vi "Pose2D_publisher.vi"() -> ()   [LabVIEW 2014]
panel:
  in  "cmdvel":T1={"msg.x"=1.01, "msg.y"=0.0, "msg.theta"=0.0}
  in  "停止":bool
  in  "发送":bool
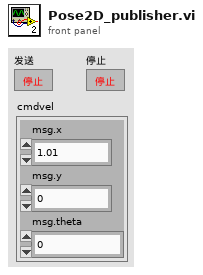
[diagram p1: front panel]
types:
  T1 = cluster{"msg.x":dbl, "msg.y":dbl, "msg.theta":dbl}
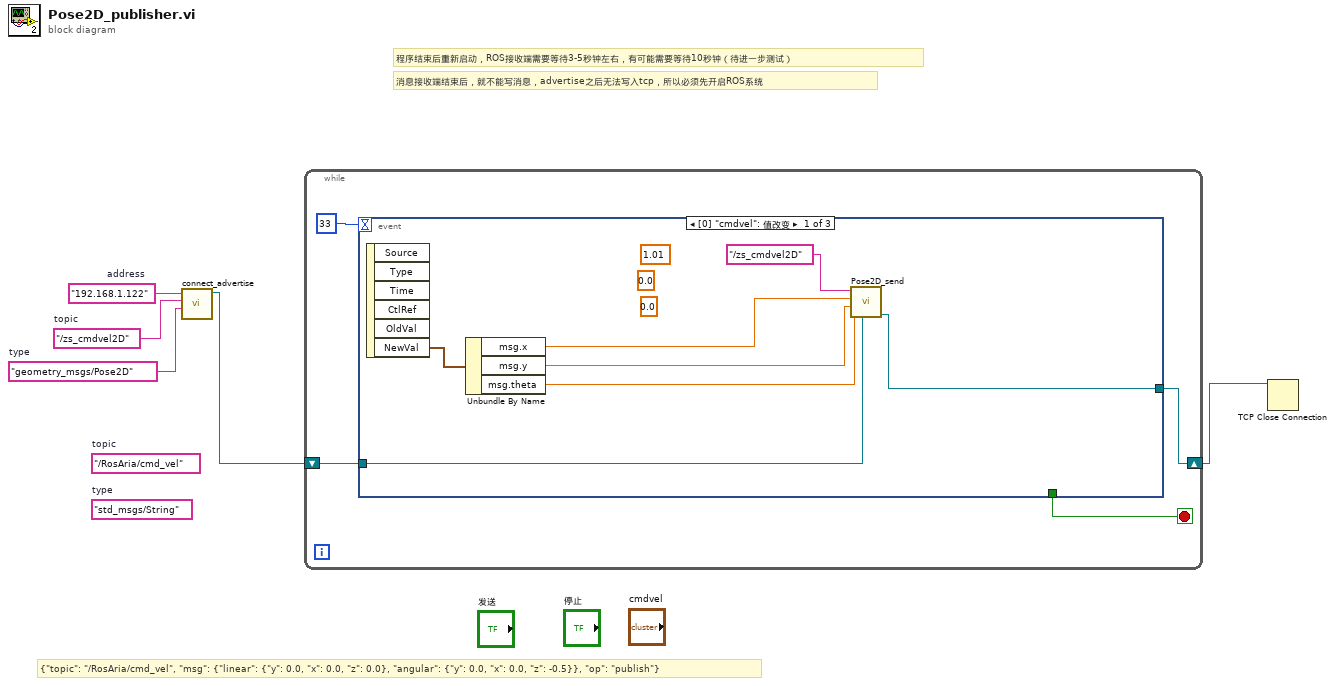
[diagram p0: block diagram]
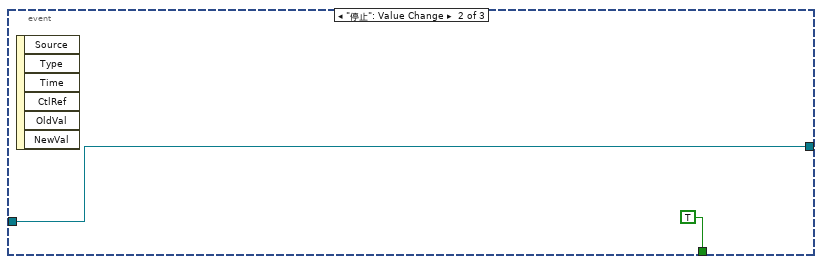
[diagram p2: hidden frame]
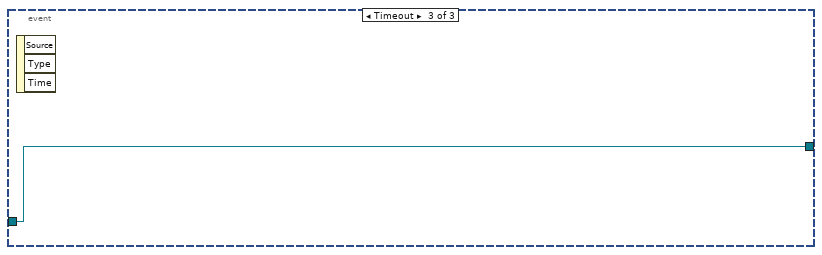
[diagram p3: hidden frame]
diagram:
  w4 = "192.168.1.122"  # address
  (unwired) "std_msgs/String"  # type
  w3 = "/zs_cmdvel2D"  # topic
  w1 = "geometry_msgs/Pose2D"  # type
  (unwired) "/RosAria/cmd_vel"  # topic
  # "消息接收端结束后，就不能写消息，advertise之后无法写入tcp，所以必须先开启ROS系统"
  # "{\"topic\": \"/RosAria/cmd_vel\", \"msg\": {\"linear\": {\"y\": 0.0, \"x\": 0.0, \"z\": 0.0}, \"angular\": {\"y\": 0.0, \"x\": 0.0, \"z\": -0.5}}, \"op\": \"publish\"}"
  # "程序结束后重新启动，ROS接收端需要等待3-5秒钟左右，有可能需要等待10秒钟（待进一步测试）"
  n1 = call "connect_advertise.vi"("type"=w1, "topic"=w3, "address"=w4) -> ("连接ID输出"=w2:refnum<k5>)  [unwired: 7 in, 1 out]
  n2 = while {
    shift-right: [w7] -> w5
    shift-left: w2 -> [w6]
    stop <- w8 stop-if-true
    n3 = event shown="[0] \"cmdvel\": 值改变" {
      selector: _ -> [_ _ _]
      dyn-events: _ -> [_ _ _]
      timeout: 33 -> [_ _ _]
      tunnel: [_ TRUE _] -> w8
      tunnel: [w10 w17 w19] -> w7
      tunnel: w6 -> [w16 w17 w19]
      event "cmdvel": Value Change {
        (unwired) 0.0 ("msg.z")
        (unwired) 0.0 ("msg.y")
        (unwired) 1.01 ("msg.x")
        n4 = event-data() -> ("NewVal"=w14:T1)  [unwired: 1 in, 5 out]
        n5 = Unbundle By Name(w14) -> ("msg.x"=w13:dbl, "msg.y"=w12:dbl, "msg.theta"=w11:dbl)
        n6 = call "Pose2D_send.vi"("连接ID"=w16, "msg.theta"=w11, "msg.y"=w12, "msg.x"=w13, "topic"="/zs_cmdvel2D") -> ("连接ID输出"=w10:refnum<k5>)  [unwired: 6 in]
      }
      event "停止": Value Change {
        n7 = event-data() -> ()  [unwired: 1 in, 6 out]
      }
      event Timeout {
        n8 = event-data() -> ()  [unwired: 1 in, 3 out]
      }
    }
  }
  n9 = TCP Close Connection(connection ID=w5) -> ()  [unwired: 2 in, 2 out]
